vi "PH_Beamline_Chief.Laser Off Activity.vi"(0 "i ref in":refnum<vi>, 2 "Laser Enabling State before":T1 items=["no info", "not disabled", "disabled"], 5 "error in":errorcluster) -> (14 "i ref out":refnum<vi>, 19 "error out":errorcluster)   [LabVIEW 2014, in "PH_Beamline_Chief.lvlib"]
uses:
  PH_Beamline_Chief.lvlib
  PH_SystemInformation/PH_SystemInformationEnabling State.ctl
  PH_Beamline/PH_Beamline.Black Box Instances.ctl
  PH_Beamline/PH_Beamline.Switch Instances.ctl
  PH_Beamline/PH_Beamline.Motion GUI Instances.ctl
  PH_Beamline/PH_Beamline.lvlib
  PH_Switch/PH_Switch.lvlib
  PH_BlackBox/PH_BlackBox.lvlib
  PH_BL-Master/PH_BL-Master.lvlib
  PH_SystemInformation/PH_SystemInformation.lvlib
  PH_Stepmotor_BaseClass/PH_Stepmotor_BaseClass.lvlib
  PH_AxisGUI_BaseClass/PH_AxisGUI_BaseClass.lvlib
  CSCore/CSSystem/CSSystemLib/CSSystemLib.lvlib
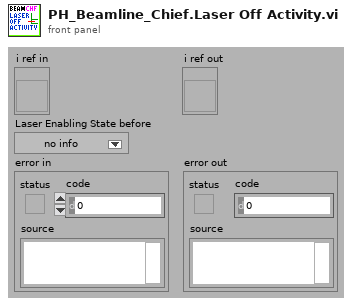
[diagram p1: front panel]
types:
  T1 = typedef "PH_SystemInformation.lvlib/PH_SystemInformationEnabling State.ctl" = i32
  T2 = enum16{"Laser", "PreAmp", "MainAmp", "Exp 1", "Exp 2", "Exp 3", "Exp 4"}
  T3 = typedef "PH_Beamline.lvlib/PH_Beamline.Motion GUI Instances.ctl" = string
  T4 = typedef "PH_Beamline.lvlib/PH_Beamline.Switch Instances.ctl" = string
  T5 = typedef "PH_Beamline.lvlib/PH_Beamline.Black Box Instances.ctl" = string
  T6 = typedef "PH_AxisGUI_BaseClass.lvlib/PH_AxisGUI_BaseClass.Database Entry.ctl" = cluster{"Address":T7, "Name":string, "Label \"Back\"":string, "Labell \"Forth\"":string}
  T7 = typedef "PH_Stepmotor_BaseClass.lvlib/PH_Stepmotor_BaseClass.Axis Address.ctl" = cluster{"Instance":string, "Motor Nr":i32}
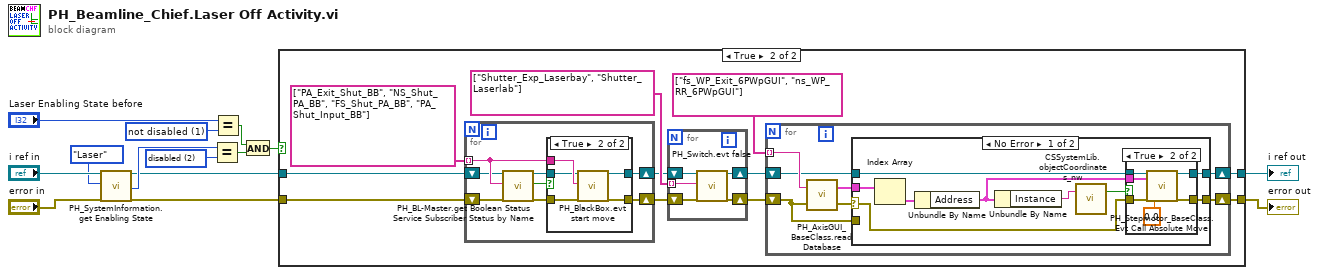
[diagram p0: block diagram]
diagram:
  w5 = T1 1 items=["no info", "not disabled", "disabled"] ("y")
  w11 = T1 2 items=["no info", "not disabled", "disabled"] ("y")
  n1 = call "PH_SystemInformation.get Enabling State.vi"("i ref in"="i ref in", "Wanted State"=T2."Laser", "error in (no error)"="error in") -> ("i ref out"=w8:refnum<vi>, "Enabling State"=w10:T1, "error out"=w6:errorcluster)  [unwired: 14 in]
  n2 = Equal?(x=w10, y=w11) -> (x = y?=w12:bool)
  n3 = Equal?(x="Laser Enabling State before", y=w5) -> (x = y?=w4:bool)
  n4 = And(x=w4, y=w12) -> (x .and. y?=w2:bool)
  n5 = case shown="True" w2 {
    tunnel: [w16 w20] -> w14
    tunnel: [w15 w21] -> w13
    tunnel: w8 -> [w16 w23]
    tunnel: w6 -> [w15 w22]
    frame False {
    }
    frame True {
      n6 = for {
        shift-right: [w65] -> w25
        shift-left: w23 -> [w63]
        shift-right: [w66] -> w24
        shift-left: w22 -> [w61]
        tunnel: T5[] ["PA_Exit_Shut_BB", "NS_Shut_PA_BB", "FS_Shut_PA_BB", "PA_Shut_Input_BB"] -> [w64] mode=indexing
        n7 = call "PH_BL-Master.get Boolean Status Service Subscriber Status by Name.vi"("i ref in"=w63, "Status Subscriber Instance"=w64, "error in (no error)"=w61) -> ("i ref out"=w62:refnum<vi>, "on/true/in?"=w59:bool, "error out"=w60:errorcluster)  [unwired: 7 in, 7 out]
        n8 = case shown="True" w59 {
          tunnel: [w67 w73] -> w66
          tunnel: [w68 w72] -> w65
          tunnel: w64 -> [_ w71]
          tunnel: w62 -> [w68 w70]
          tunnel: w60 -> [w67 w69]
          frame False {
          }
          frame True {
            n9 = call "PH_BlackBox.evt start move.vi"("i ref in"=w70, "Instance"=w71, "error in (no error)"=w69) -> ("i ref out"=w72:refnum<vi>, "error out"=w73:errorcluster)  [unwired: 15 in]
          }
        }
      }
      n10 = for {
        shift-right: [w57] -> w17
        shift-left: w25 -> [w55]
        shift-right: [w58] -> w19
        shift-left: w24 -> [w54]
        tunnel: T4[] ["Shutter_Exp_Laserbay", "Shutter_Laserlab"] -> [w56] mode=indexing
        n11 = call "PH_Switch.evt false.vi"("i ref in"=w55, "Instance"=w56, "error in (no error)"=w54) -> ("i ref out"=w57:refnum<vi>, "error out"=w58:errorcluster)  [unwired: 15 in]
      }
      n12 = for {
        tunnel: T3[] ["fs_WP_Exit_6PWpGUI", "ns_WP_RR_6PWpGUI"] -> [w32] mode=indexing
        shift-right: [w34] -> w21
        shift-left: w19 -> [w29]
        shift-right: [w33] -> w20
        shift-left: w17 -> [w31]
        n13 = call "PH_AxisGUI_BaseClass.read Database.vi"("error in (no error)"=w29, "DB Entry to read"=w32) -> ("error out"=w30:errorcluster, "DB EntriesArray"=w28:T6[])
        n14 = case shown="No Error" w30 {
          selector: w30 -> [w35 _]
          tunnel: [w43 w53] -> w34
          tunnel: [w42 w52] -> w33
          tunnel: w31 -> [w41 w52]
          tunnel: w29 -> [_ w53]
          tunnel: w28 -> [w40 _]
          frame No Error {
            n15 = Index Array(array=w40) -> (element=w39:T6)  [unwired: 1 in]
            n16 = Unbundle By Name(w39) -> ("Address"=w38:T7)
            n17 = Unbundle By Name(w38) -> ("Instance"=w37:string)
            n18 = call "CSSystemLib.objectCoordinates_nw.vi"("name"=w37) -> ("obj exists"=w36:bool)  [unwired: 15 in, 3 out]
            n19 = case shown="True" w36 {
              tunnel: [w44 w51] -> w43
              tunnel: [w45 w50] -> w42
              tunnel: w41 -> [w45 w49]
              tunnel: w35 -> [w44 w47]
              tunnel: w38 -> [_ w46]
              frame False {
              }
              frame True {
                n20 = call "PH_Stepmotor_BaseClass.Evt Call Absolute Move.vi"("i ref in"=w49, "Address"=w46, "error in"=w47, "Target Position (Units)"=0.0) -> ("i ref out"=w50:refnum<vi>, "error out"=w51:errorcluster)  [unwired: 14 in]
              }
            }
          }
          frame Error {
          }
        }
      }
    }
  }
  "error out" <- w13
  "i ref out" <- w14
